vi "Team and Side.vi"(9 "Field Size 2":T4, 10 "Game Status":T6 {"Time" format="%<%.3X %x>T"; "Blue Timeout Remaining" format="%<%M:%S>t"; "Yellow Timeout Remaining" format="%<%M:%S>t"; "Time Left" format="%<%M:%S>t"}, 11 "Input Detection Frame":T9) -> (3 "Output IA Input":T1)   [LabVIEW 2016]
uses:
  SSL Detection Robot.ctl
  SSL Detection Ball.ctl
  SSL Referee Game Status.ctl
  Field Size.ctl
  AI Input.ctl
  AI Robot.ctl
  AI Ball.ctl
  AI Judge.ctl
panel:
  in  "Lado":enum16{"Esquerdo", "Direito"}(ring) caption="Enum"
  in  "Time":enum16{"Azul", "Amarelo"}(ring) caption="Enum"
  # "Score"
  # "Red Cards"
  # "Yellow Cards"
  # "Timeouts Left"
  # "Timeout Remaining"
  # "Goalie ID"
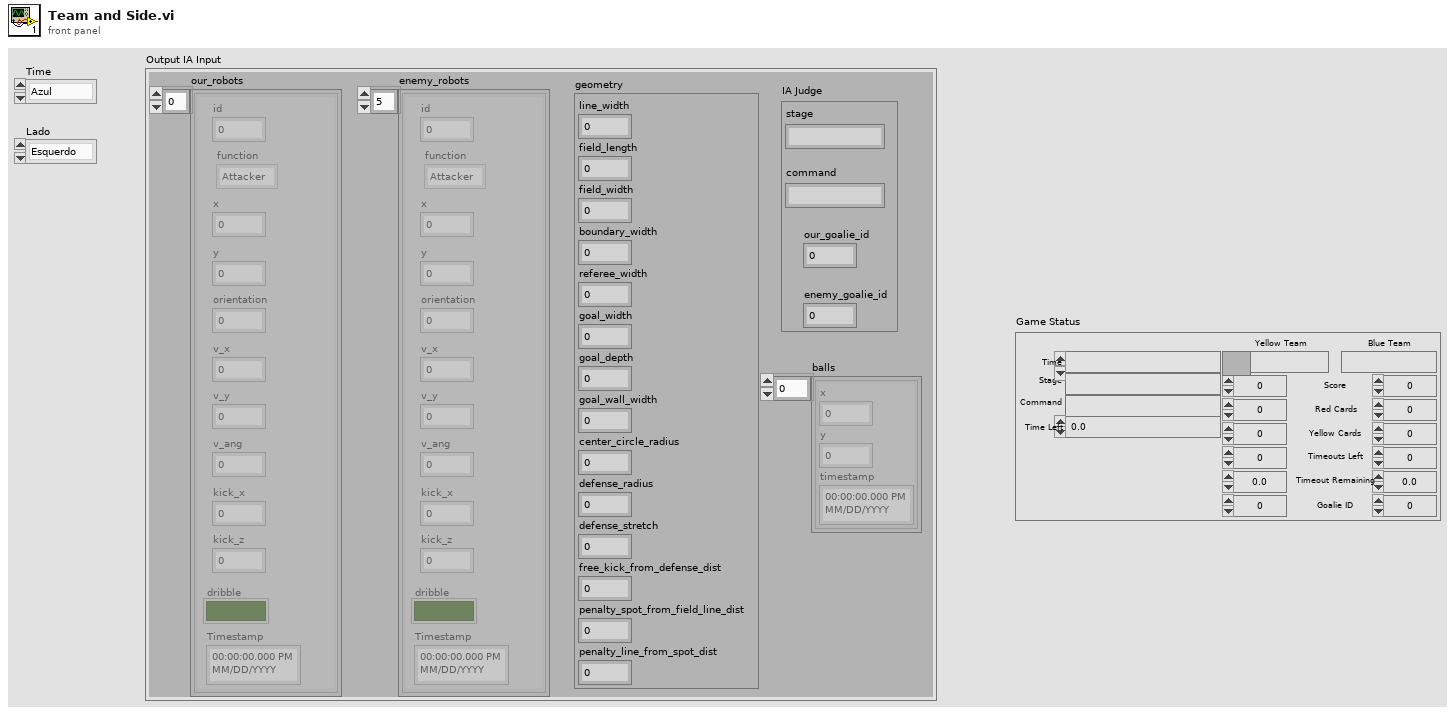
[diagram p1: front panel]
types:
  T1 = typedef "AI Input.ctl" = cluster{"our_robots":T2[], "enemy_robots":T2[], "balls":T3[], "geometry":T4, "IA Judge":T5}
  T2 = typedef "AI Robot.ctl" = cluster{"id":u32, "function":enum16{"Attacker", "Goalie", "Defender"}, "x":dbl, "y":dbl, "orientation":dbl, "v_x":dbl, "v_y":dbl, "v_ang":dbl, "kick_x":dbl, "kick_z":dbl, "dribble":bool, "Timestamp":timestamp}
  T3 = typedef "AI Ball.ctl" = cluster{"x":dbl, "y":dbl, "timestamp":timestamp}
  T4 = typedef "Field Size.ctl" = cluster{"line_width":u32, "field_length":u32, "field_width":u32, "boundary_width":u32, "referee_width":u32, "goal_width":u32, "goal_depth":u32, "goal_wall_width":u32, "center_circle_radius":u32, "defense_radius":u32, "defense_stretch":u32, "free_kick_from_defense_dist":u32, "penalty_spot_from_field_line_dist":u32, "penalty_line_from_spot_dist":u32}
  T5 = typedef "AI Judge.ctl" = cluster{"stage":string, "command":string, "our_goalie_id":dbl, "enemy_goalie_id":dbl}
  T6 = typedef "SSL Referee Game Status.ctl" = cluster{"Stage":string, "Command":string, "Time Left":dbl, "Yellow Team":string, "Blue Team":string, "Yellow Score":u32, "Blue Score":u32, "Yellow Red Cards":u32, "Blue Red Cards":u32, "Yellow Yellow Cards":u32, "Blue Yellow Cards":u32, "Yellow Timeouts Left":u32, "Blue Timeouts Left":u32, "Yellow Timeout Remaining":dbl, "Blue Timeout Remaining":dbl, "Yellow Goalie Id":u32, "Blue Goalie Id":u32, "Time":timestamp}
  T7 = typedef "SSL Detection Robot.ctl" = cluster{"x":dbl, "robot_id":u32, "confidence":sgl, "y":sgl, "orientation":sgl, "pixel_x":sgl, "pixel_y":sgl, "height":sgl, "Valid":bool, "Time Stamp":timestamp}
  T8 = typedef "SSL Detection Ball.ctl" = cluster{"x":sgl, "area":u32, "confidence":sgl, "y":sgl, "z":sgl, "pixel_x":sgl, "pixel_y":sgl, "Valid":bool, "Time Stamp":timestamp}
  T9 = cluster{"frame_number":u32, "t_capture":dbl, "t_sent":dbl, "camera_id":u32, "robots_yellow":T7[], "robots_blue":T7[], "balls":T8[], "Valid":bool, "Time Stamp":timestamp}
  T10 = typedef "SSL Detection Frame.ctl" = cluster{"frame_number":u32, "t_capture":dbl, "t_sent":dbl, "camera_id":u32, "robots_yellow":T7[], "robots_blue":T7[], "balls":T8[], "Valid":bool, "Time Stamp":timestamp}
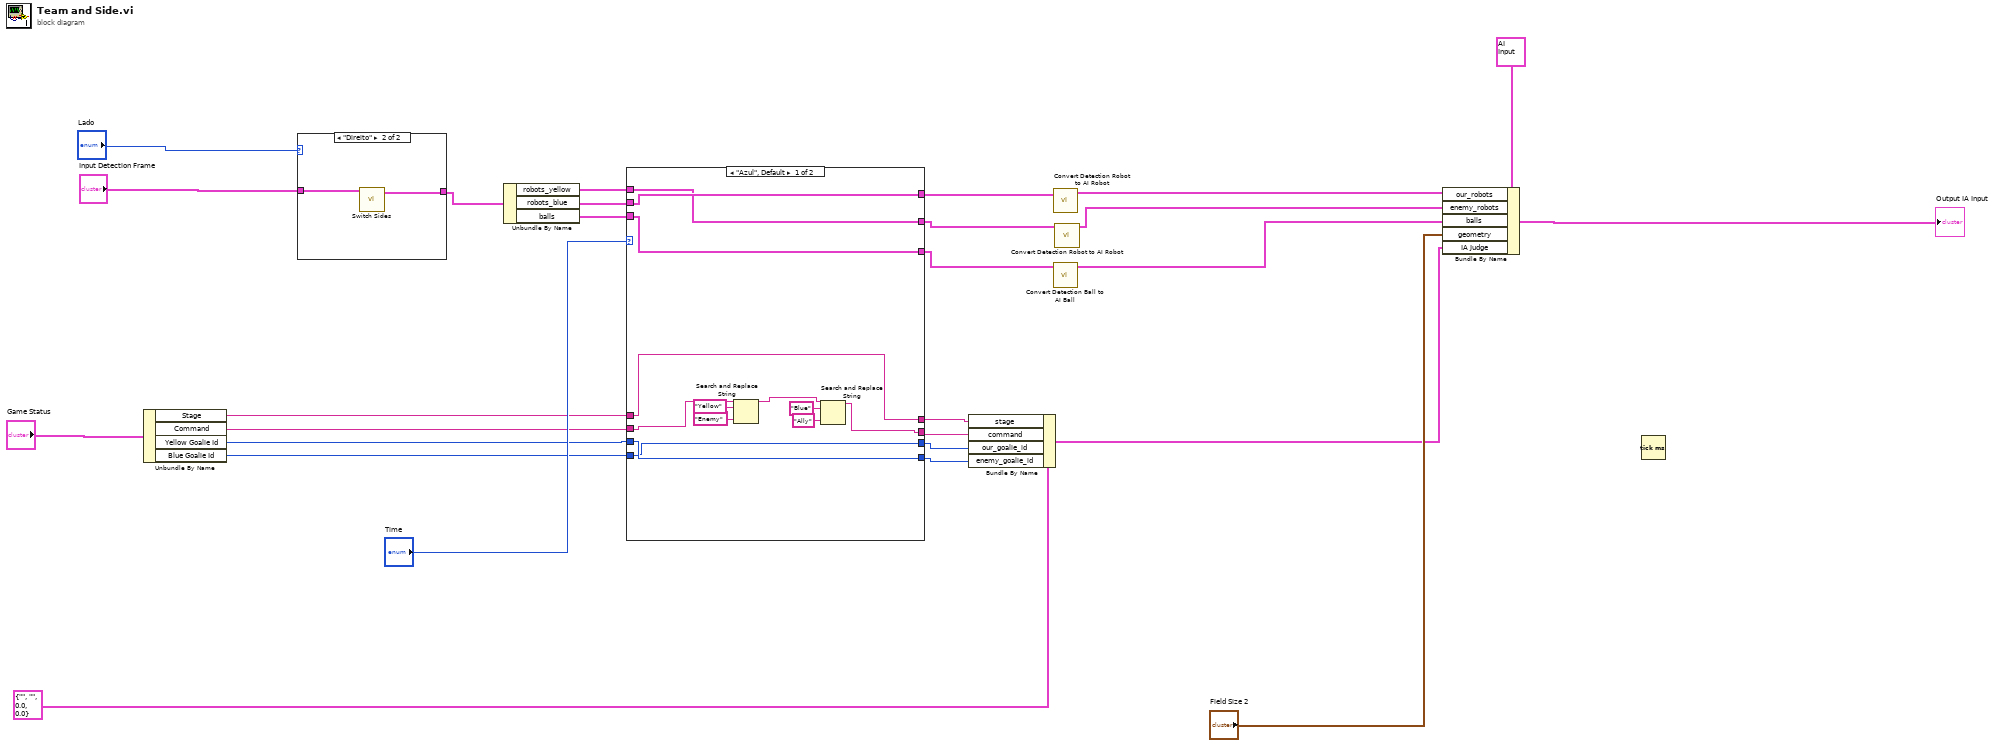
[diagram p0: block diagram]
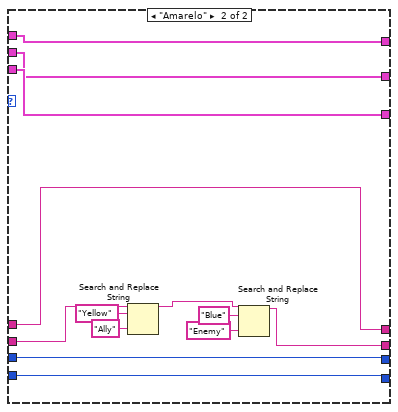
[diagram p2: hidden frame]
diagram:
  n1 = Unbundle By Name("Game Status") -> ("Stage"=w12:string, "Command"=w11:string, "Yellow Goalie Id"=w16:u32, "Blue Goalie Id"=w15:u32)
  n2 = case shown="\"Direito\"" "Lado" {
    tunnel: "Input Detection Frame" -> [w28 w30]
    tunnel: [w28 w29] -> w23
    frame "Esquerdo", Default {
    }
    frame "Direito" {
      n3 = call "Switch Sides.vi"("Detection Frame"=w30) -> ("output cluster"=w29:T10)  [unwired: 10 in]
    }
  }
  n4 = Unbundle By Name(w23) -> ("robots_yellow"=w22:T7[], "robots_blue"=w21:T7[], "balls"=w20:T8[])
  n5 = case shown="\"Azul\", Default" "Time" {
    tunnel: w22 -> [w42 w54]
    tunnel: w21 -> [w43 w55]
    tunnel: w20 -> [w41 w56]
    tunnel: [w43 w54] -> w6
    tunnel: [w42 w55] -> w4
    tunnel: [w41 w56] -> w2
    tunnel: w16 -> [w40 w53]
    tunnel: w15 -> [w39 w52]
    tunnel: [w40 w52] -> w9
    tunnel: [w39 w53] -> w10
    tunnel: w12 -> [w31 w51]
    tunnel: w11 -> [w33 w50]
    tunnel: [w31 w51] -> w8
    tunnel: [w32 w44] -> w7
    frame "Azul", Default {
      n6 = Search and Replace String(input string=w33, search string="Yellow", replace string="Enemy" ("replace string (\"\")")) -> (result string=w38:string)  [unwired: 5 in, 3 out]
      n7 = Search and Replace String(input string=w38, search string="Blue", replace string="Ally" ("replace string (\"\")")) -> (result string=w32:string)  [unwired: 5 in, 3 out]
    }
    frame "Amarelo" {
      n8 = Search and Replace String(input string=w50, search string="Yellow", replace string="Ally" ("replace string (\"\")")) -> (result string=w45:string)  [unwired: 5 in, 3 out]
      n9 = Search and Replace String(input string=w45, search string="Blue", replace string="Enemy" ("replace string (\"\")")) -> (result string=w44:string)  [unwired: 5 in, 3 out]
    }
  }
  n10 = Bundle By Name(cluster=T5 {"stage"="", "command"="", "our_goalie_id"=0.0, "enemy_goalie_id"=0.0} ("IA Judge"), "stage"=w8, "command"=w7, "our_goalie_id"=w10, "enemy_goalie_id"=w9) -> (w14:T5)
  n11 = call "Convert Detection Robot to AI Robot.vi"("Input"=w6) -> ("Output"=w5:T2[])  [unwired: 10 in]
  n12 = call "Convert Detection Ball to AI Ball.vi"("Input"=w2) -> ("Output"=w1:T3[])  [unwired: 10 in]
  n13 = call "Convert Detection Robot to AI Robot.vi"("Input"=w4) -> ("Output"=w3:T2[])  [unwired: 10 in]
  n14 = Bundle By Name(cluster=T1 {"our_robots"=[], "enemy_robots"=[], "balls"=[], "geometry"={"line_width"=0, "field_length"=0, "field_width"=0, "boundary_width"=0, "referee_width"=0, "goal_width"=0, "goal_depth"=0, "goal_wall_width"=0, "center_circle_radius"=0, "defense_radius"=0, "defense_stretch"=0, "free_kick_from_defense_dist"=0, "penalty_spot_from_field_line_dist"=0, "penalty_line_from_spot_dist"=0}, "IA Judge"={"stage"="", "command"="", "our_goalie_id"=0.0, "enemy_goalie_id"=0.0}} ("Detection Frame"), "our_robots"=w5, "enemy_robots"=w3, "balls"=w1, "geometry"="Field Size 2", "IA Judge"=w14) -> (→"Output IA Input":T1)
  n15 = Tick Count (ms)() -> ()  [unwired: 1 out]
